vi "oa_Align Vibration Signals with Tach Pulses.vi"(7 "reset? (True)":bool=TRUE, 9 "remaining delay length":i32, 10 "deleted portion":dbl[](array[numeric]) format="%.2f", 11 "scaled signals (EU) in":waveform(dbl)[](array[waveform])) -> (1 "# of delayed samples":dbl, 3 "scaled signals (EU) out":waveform(dbl)[](array[waveform]))   [LabVIEW 2017, in "SoundVib_Resampling.lvlib"]
uses:
  <vilib>/addons/Sound and Vibration/Order Analysis/Resample Order Tracking/SoundVib_Resampling.lvlib
panel:
  in  "empty waveform":waveform(dbl)
  in  "empty waveform array":waveform(dbl)[](array[waveform])
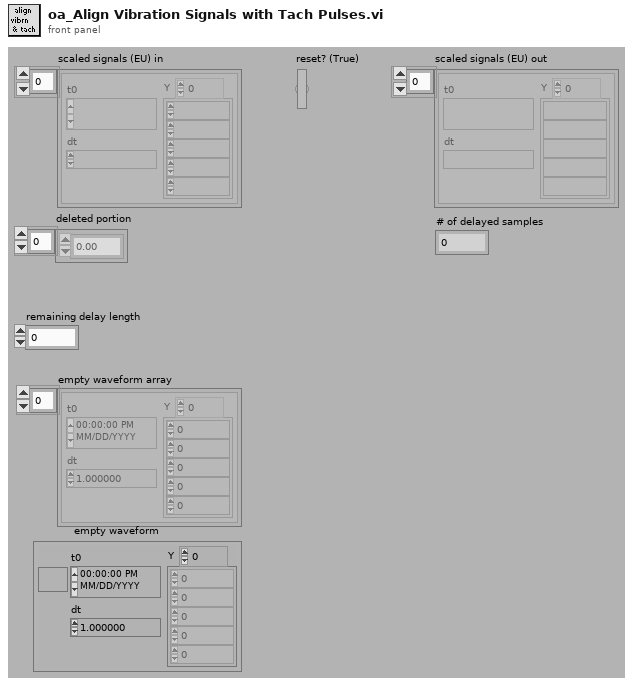
[diagram p1: front panel]
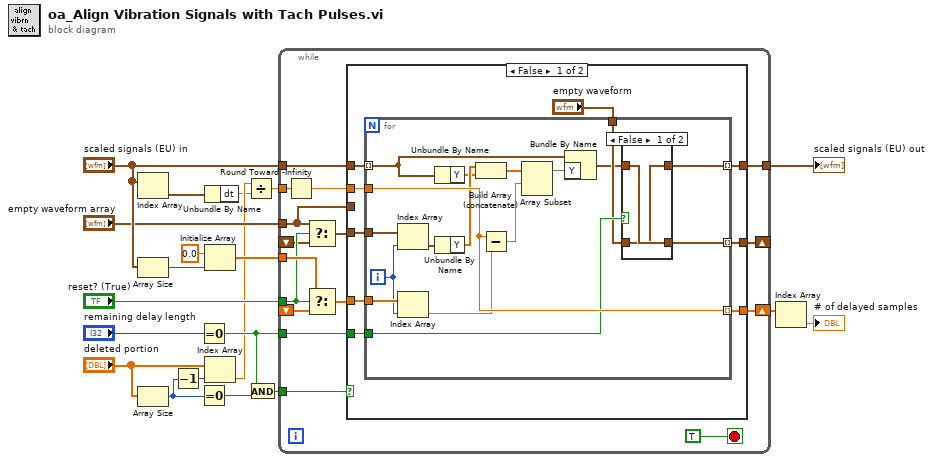
[diagram p0: block diagram]
diagram:
  n1 = Index Array(array="scaled signals (EU) in") -> (element=w16:waveform(dbl))  [unwired: 1 in]
  n2 = Array Size(array="scaled signals (EU) in") -> (size(s)=w13:i32)
  n3 = Array Size(array="deleted portion") -> (size(s)=w18:i32)
  n4 = Decrement(x=w18) -> (x-1=w17:i32)
  n5 = Equal To 0?(x="remaining delay length") -> (x = 0?=w7:bool)
  n6 = Equal To 0?(x=w18) -> (x = 0?=w6:bool)
  n7 = Unbundle By Name(w16) -> ("dt"=w4:dbl)
  n8 = Initialize Array(0.0 ("element"), w13) -> (w11:dbl[])
  n9 = Index Array(array="deleted portion", index=w17) -> (element=w5:dbl)
  n10 = Divide(x=w5, y=w4) -> (x/y=w10:dbl)
  n11 = And(x=w7, y=w6) -> (x .and. y?=w3:bool)
  n12 = while {
    shift-right: [w30] -> w2
    shift-left: _ -> [w34]
    tunnel: "scaled signals (EU) in" -> [w35]
    tunnel: "reset? (True)" -> [w26]
    tunnel: w11 -> [w32]
    tunnel: w10 -> [w31]
    tunnel: [w29] -> w20
    tunnel: w7 -> [w28]
    shift-right: [w27] -> _
    shift-left: _ -> [w25]
    tunnel: "empty waveform array" -> [w22]
    tunnel: w3 -> [w23]
    stop <- TRUE stop-if-true
    n13 = Round Toward -Infinity(1:w31) -> (0:w21:dbl)
    n14 = Select(t=w22, s=w26, f=w25) -> (s? t:f=w24:waveform(dbl)[])
    n15 = Select(t=w32, s=w26, f=w34) -> (s? t:f=w33:dbl[])
    n16 = case shown="False" w23 {
      tunnel: w35 -> [w45 w69]
      tunnel: w33 -> [w44 w67]
      tunnel: w21 -> [w43 _]
      tunnel: [w42 w67] -> w30
      tunnel: [w41 w69] -> w29
      tunnel: w28 -> [w40 _]
      tunnel: [w39 w68] -> w27
      tunnel: w24 -> [w38 _]
      tunnel: w22 -> [_ w68]
      frame False {
        n17 = for {
          tunnel: w45 -> [w52] mode=indexing
          tunnel: w44 -> [w57]
          tunnel: w43 -> [w62]
          tunnel: [w62] -> w42 mode=indexing
          tunnel: [w60] -> w41 mode=indexing
          tunnel: w40 -> [w61]
          tunnel: [w59] -> w39 mode=indexing
          tunnel: w38 -> [w58]
          tunnel: "empty waveform" -> [w54]
          i -> [w56]
          n18 = Index Array(array=w58, index=w56) -> (element=w53:waveform(dbl))
          n19 = Index Array(array=w57, index=w56) -> (element=w55:dbl)
          n20 = Unbundle By Name(w52) -> ("Y"=w50:dbl[])
          n21 = Unbundle By Name(w53) -> ("Y"=w51:dbl[])
          n22 = Build Array (concatenate)(w51, w50) -> (w47:dbl[])
          n23 = Subtract(x=w62, y=w55) -> (x-y=w48:dbl)
          n24 = Array Subset(array=w47, index=w48) -> (w46:dbl[])  [unwired: 1 in]
          n25 = Bundle By Name(cluster=w52, "Y"=w46) -> (w49:waveform(dbl))
          n26 = case shown="False" w61 {
            tunnel: w49 -> [w64 w66]
            tunnel: [w63 w66] -> w60
            tunnel: [w64 w65] -> w59
            tunnel: w54 -> [w63 w65]
            frame False {
            }
            frame True {
            }
          }
        }
      }
      frame True {
      }
    }
  }
  "scaled signals (EU) out" <- w20
  n27 = Index Array(array=w2) -> (element=→"# of delayed samples":dbl)  [unwired: 1 in]
